vi "Set Settings.vi"(10 "settings":T1, 11 "Configuration in":refnum<class "Configuration.lvclass">) -> (3 "Configuration out":refnum<class "Configuration.lvclass">)   [LabVIEW 2017, in "Data Sharing Framework Core.lvlib" / "Data Sharing Framework Engine.lvlib" / "Configuration.lvclass"]
uses:
  Configuration.lvclass
  Configuration/1.0.0/Public/Controls/DSF Settings Info.ctl
  Configuration.lvclass/Configuration.ctl
  Configuration/1.0.0/Data Sharing Framework Configuration.lvlib
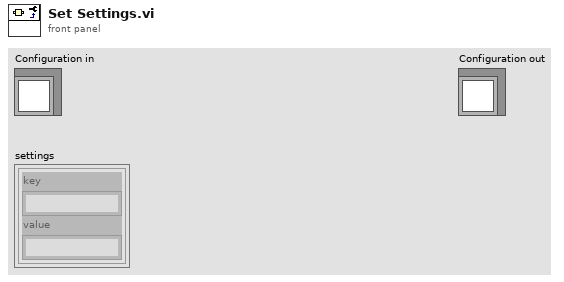
[diagram p1: front panel]
types:
  T1 = typedef "Data Sharing Framework Core.lvlib/Data Sharing Framework Configuration.lvlib/DSF Settings Info.ctl" = cluster{"key":string, "value":string}[]
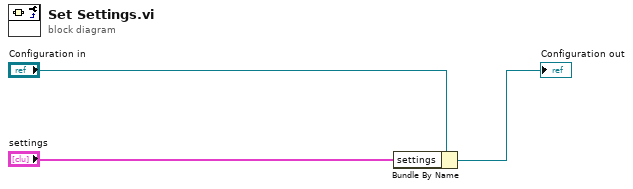
[diagram p0: block diagram]
diagram:
  n1 = Bundle By Name(cluster="Configuration in", "settings"="settings") -> (→"Configuration out":refnum<class "Configuration.lvclass">)
